vi "Plot Editor_Plot to Data & Controls.vi"(6 "Control Refnums":refnum<vi>[](array[refnum]), 7 "XYGraph in":refnum<vi>, 8 "error in (no error)":errorcluster, 11 "Plot Editor Internal Data in":T1) -> (0 "error out":errorcluster, 3 "Plot Editor Internal Data out":T1)   [LabVIEW 2021, in "Plot Editor.lvlib"]
uses:
  Plot Editor.lvlib
  Plot Editor Internal Variables.ctl
  XY Graph/XY Graph Plot Properties.ctl
  XY Graph/XY Graph Add-Ons.lvlib
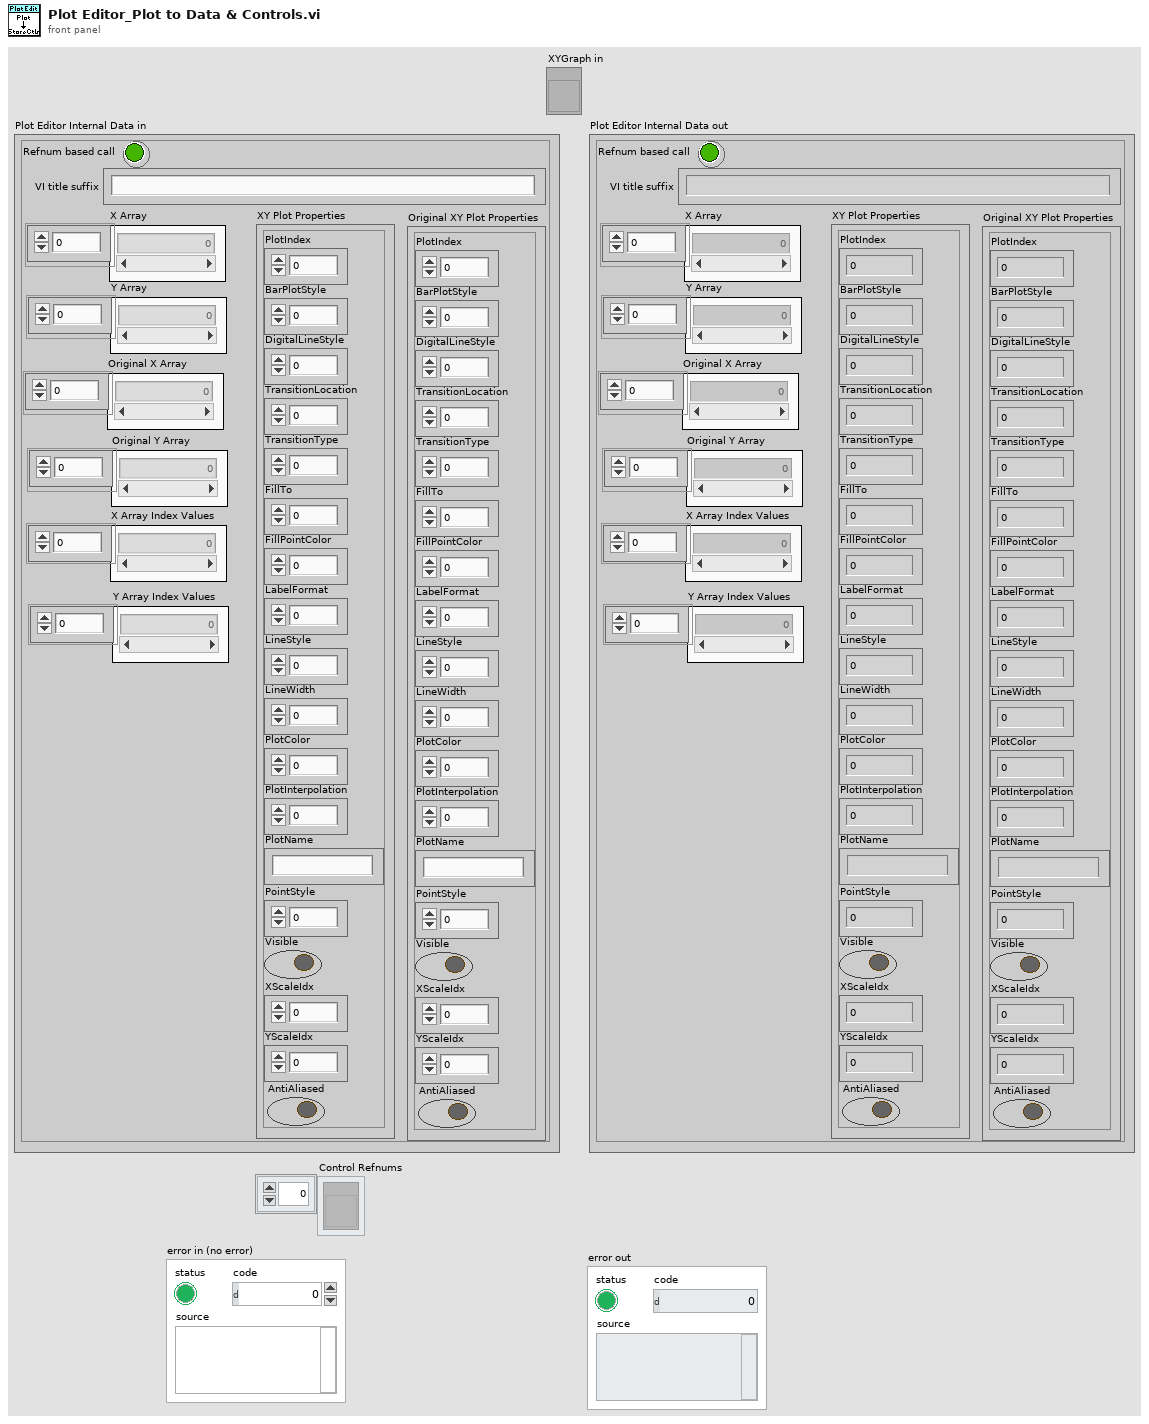
[diagram p1: front panel]
types:
  T1 = typedef "Plot Editor.lvlib/Plot Editor Internal Variables.ctl" = cluster{"X Array":dbl[], "Y Array":dbl[], "XY Plot Properties":T2, "X Array Index Values":u32[], "Y Array Index Values":u32[], "Original XY Plot Properties":T2, "Original X Array":dbl[], "Original Y Array":dbl[], "VI title suffix":string, "Refnum based call":bool}
  T2 = typedef "XY Graph Add-Ons.lvlib/XY Graph Plot Properties.ctl" = cluster{"PlotIndex":i32, "BarPlotStyle":u8, "DigitalLineStyle":u8, "TransitionLocation":u8, "TransitionType":u8, "FillTo":i16, "FillPointColor":u32, "LabelFormat":u8, "LineStyle":u8, "LineWidth":u8, "PlotColor":u32, "PlotInterpolation":u8, "PlotName":string, "PointStyle":u8, "Visible":bool, "XScaleIdx":u32, "YScaleIdx":u32, "AntiAliased":bool}
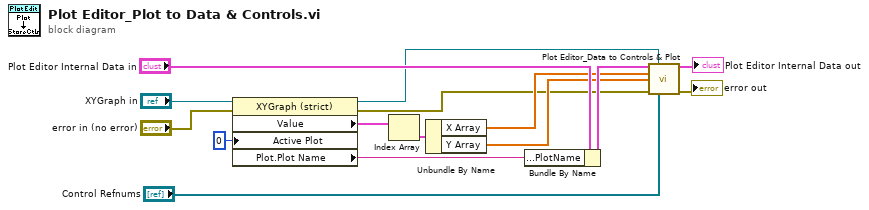
[diagram p0: block diagram]
diagram:
  n1 = property class="XYGraph (strict)"(reference="XYGraph in", error in="error in (no error)", "Active Plot"=u32 0) -> (reference out=w5:refnum<vi>, error out=w3:errorcluster, "Value"=w12:cluster{"X Array":dbl[], "Y Array":dbl[]}[], "Plot.Plot Name"=w9:string)
  n2 = Index Array(array=w12) -> (element=w11:cluster{"X Array":dbl[], "Y Array":dbl[]})  [unwired: 1 in]
  n3 = Unbundle By Name(w11) -> ("X Array"=w7:dbl[], "Y Array"=w6:dbl[])
  n4 = Bundle By Name(cluster="Plot Editor Internal Data in", "XY Plot Properties.PlotName"=w9) -> (w8:T1)
  n5 = call "Plot Editor_Data to Controls & Plot.vi"("Plot Editor Internal Data"=w8, "XYGraph in"=w5, "X Array"=w7, "Y Array"=w6, "error in (no error)"=w3, "Control Refnums"="Control Refnums") -> ("Plot Editor Internal Data"=→"Plot Editor Internal Data out":T1, "error out"=→"error out":errorcluster)  [unwired: 8 in]
